vi "write_resolution_attributes.vi"(8 "error in (no error)":errorcluster, 10 "resolution":dbl format="%#_13g", 11 "HDF5 Ref":T1) -> (0 "error out":errorcluster, 3 "HDF5 Ref out":T1)   [LabVIEW 2015, in "hdf5_photon_record_log.lvclass"]
uses:
  hdf5_photon_record_log.lvclass
  <vilib>/UPVI/lvhdf5/library.llb/HDF5 Ref.ctl
  <vilib>/UPVI/lvhdf5/attribute.llb/Simple H5Awrite (Variant).vi
  <vilib>/UPVI/lvhdf5/attribute.llb/LVH5A Operation.ctl
  <vilib>/UPVI/lvhdf5/attribute.llb/Simple H5Awrite.xnode
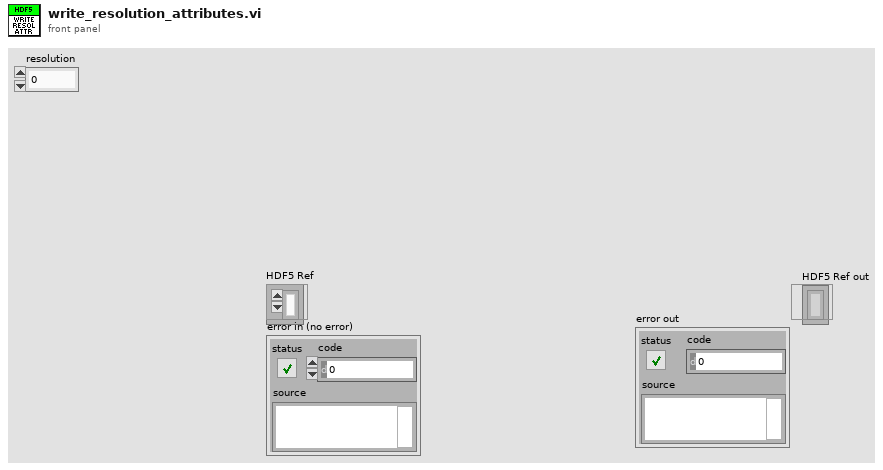
[diagram p1: front panel]
types:
  T1 = typedef "HDF5 Ref.ctl" = refnum<k1>
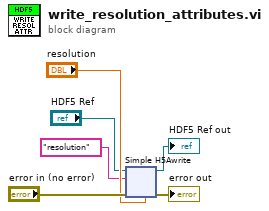
[diagram p0: block diagram]
diagram:
  n1 = xnode "Simple H5Awrite"("HDF5 Ref"="HDF5 Ref", "Name"="resolution", "error in (no error)"="error in (no error)", "Value"="resolution") -> ("HDF5 Ref out"=→"HDF5 Ref out":T1, "error out"=→"error out":errorcluster)  [unwired: 1 in]
